vi "Load by Identifier.vi"(8 "error in (no error)":errorcluster, 10 "Identifier":string, 11 "User Provider in":refnum<class "User Provider.lvclass">) -> (0 "error out":errorcluster, 2 "User":refnum<class "User.lvclass">, 3 "User Provider out":refnum<class "User Provider.lvclass">)   [LabVIEW 2020, in "HTTP Server.lvlib" / "User Provider.lvclass"]
uses:
  User Provider.lvclass
  User/User.lvclass
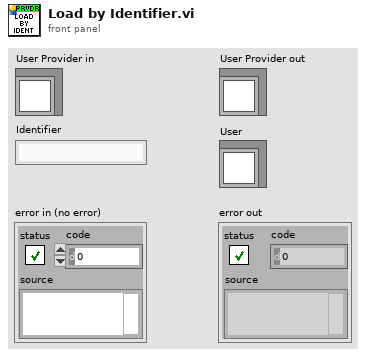
[diagram p1: front panel]
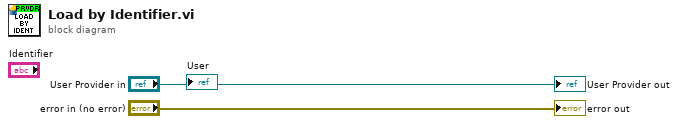
[diagram p0: block diagram]
diagram:
  "error out" <- "error in (no error)"
  "User Provider out" <- "User Provider in"
